vi "Compute_Intersection_2_Lines.vi"(8 "m'":sgl, 9 "b'":sgl, 10 "b":sgl, 11 "m":sgl) -> (2 "Yint":sgl, 3 "Xint":sgl)   [LabVIEW 2015]
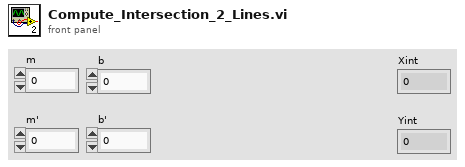
[diagram p1: front panel]
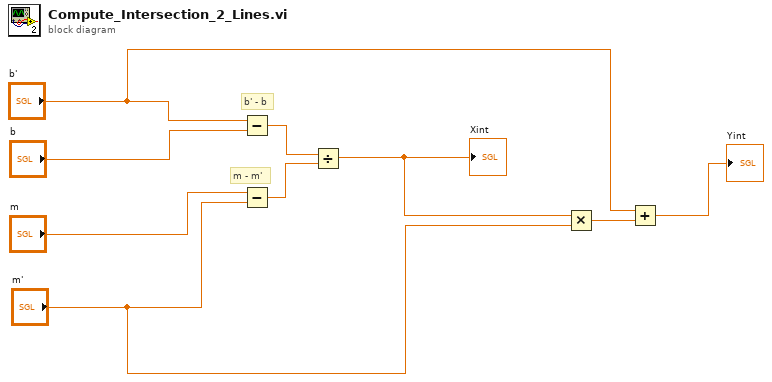
[diagram p0: block diagram]
diagram:
  # "m - m'"
  # "b' - b"
  n1 = Subtract(x="b'", y="b") -> (x-y=w8:sgl)
  n2 = Subtract(x="m", y="m'") -> (x-y=w7:sgl)
  n3 = Divide(x=w8, y=w7) -> (x/y=w3:sgl)
  "Xint" <- w3
  n4 = Multiply(x=w3, y="m'") -> (x*y=w4:sgl)
  n5 = Add(x="b'", y=w4) -> (x+y=→"Yint":sgl)
